vi "MouseInDrawArea.vi"(9 "Coords":T1, 10 "XYGraph输入":refnum<vi>) -> (1 "InOrNot":bool, 2 "XY":cluster{"X":dbl, "Y":dbl})   [LabVIEW 2015]
uses:
  <vilib>/Utility/miscctls.llb/LVPoint32TypeDef.ctl
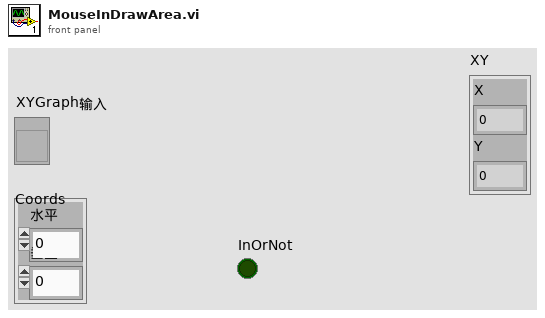
[diagram p1: front panel]
types:
  T1 = typedef "LVPoint32TypeDef.ctl" = cluster{"Horizontal":i32, "Vertical":i32}
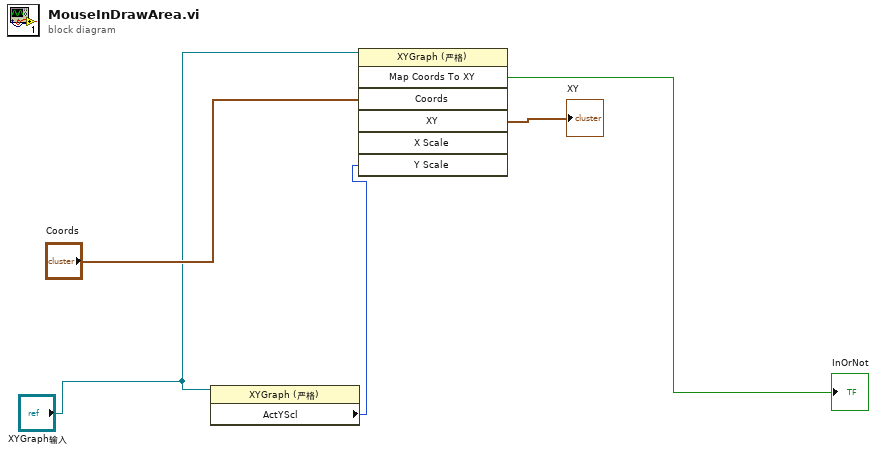
[diagram p0: block diagram]
diagram:
  n1 = property class="XYGraph (严格)"(reference="XYGraph输入") -> ("ActYScl"=w1:i32)  [unwired: 1 in, 2 out]
  n2 = invoke class="XYGraph (严格)" method="Map Coords To XY"(reference="XYGraph输入", "Coords"="Coords", "Y Scale"=w1) -> ("Map Coords To XY"=→"InOrNot":bool, "XY"=→"XY":cluster{"X":dbl, "Y":dbl})  [unwired: 4 in, 5 out]
